vi "analyze graph array.vi"(7 "appended graphs":bool=TRUE, 9 "plot# per file":u16[](array[numeric])=[3, 1], 10 "column extension":string[](array[string])=["046", "044", "042"], 11 "graph file":cluster{"all rows":dbl[], "all rows":dbl[]}[](array[cluster])) -> (0 "total plot# per file":u16, 2 "reshuffled graph file":cluster{"all rows":dbl[], "all rows":dbl[]}[](array[cluster]), 3 "graph array summary":cluster{"index":u16, "length":u16}[](array[cluster]))   [LabVIEW 2025]
panel:
  out "valid":bool
  # "Find patterns of XY graphs\nInput: XY graphs from multiple data files. Each data file may have multiple plots. \nThe plots consists of singleX-multipleY and singleX-single Y and so forth.\n\n(1) Count number of the datafiles (same with the number of column extension)\n(2) Extract XY graphs of a single datafile, whose patterns are repeated for entire data files.\n(3) From the extracted XY graphs,  count number of rows of each xy-graph and find patterns\nin terms of the same number of rows (possibly due to graphs of same x-axis)."
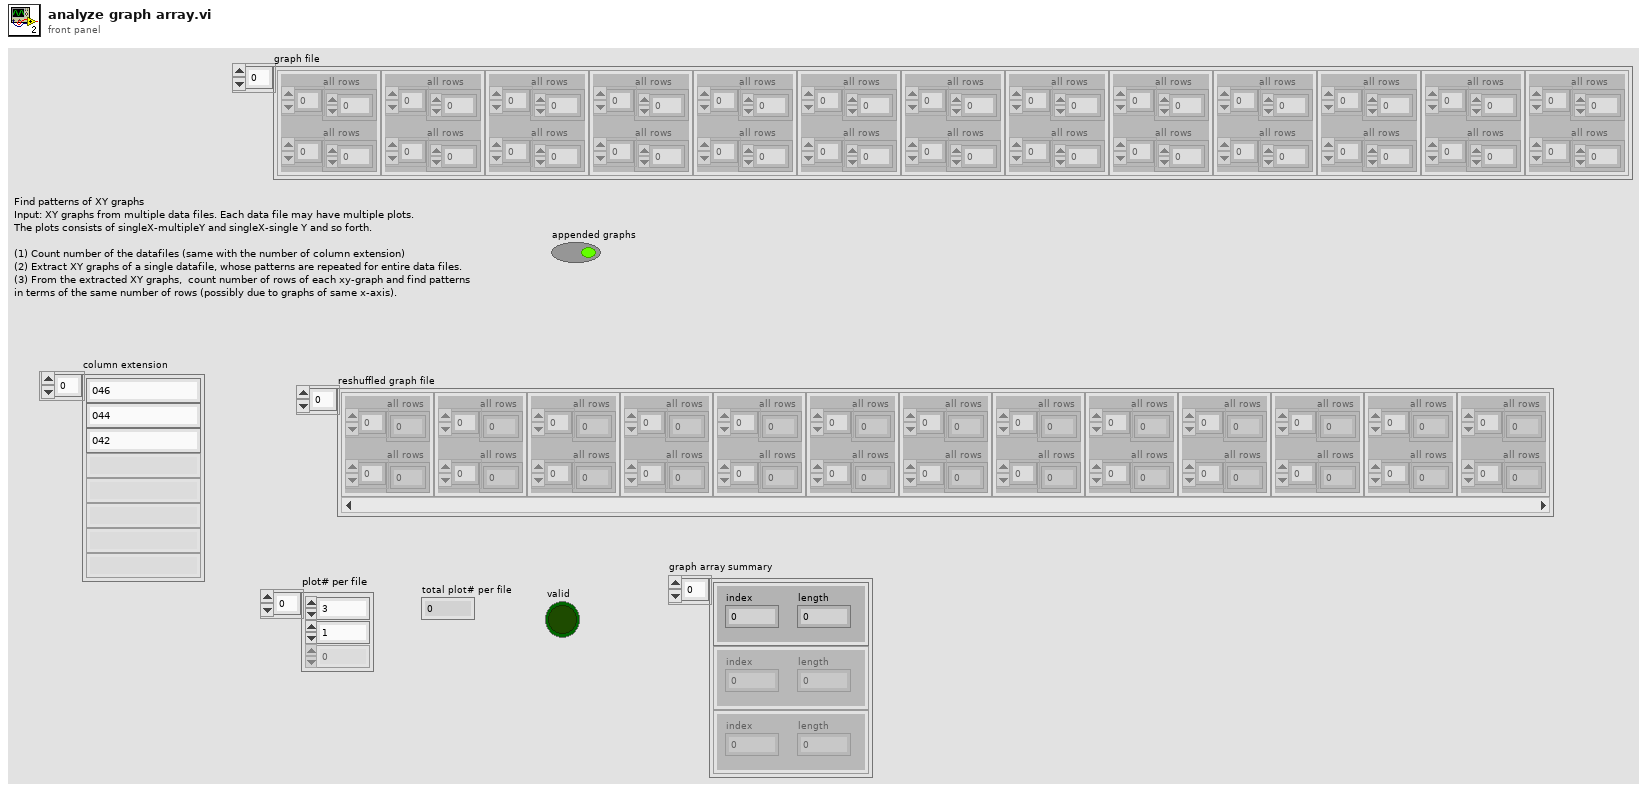
[diagram p1: front panel]
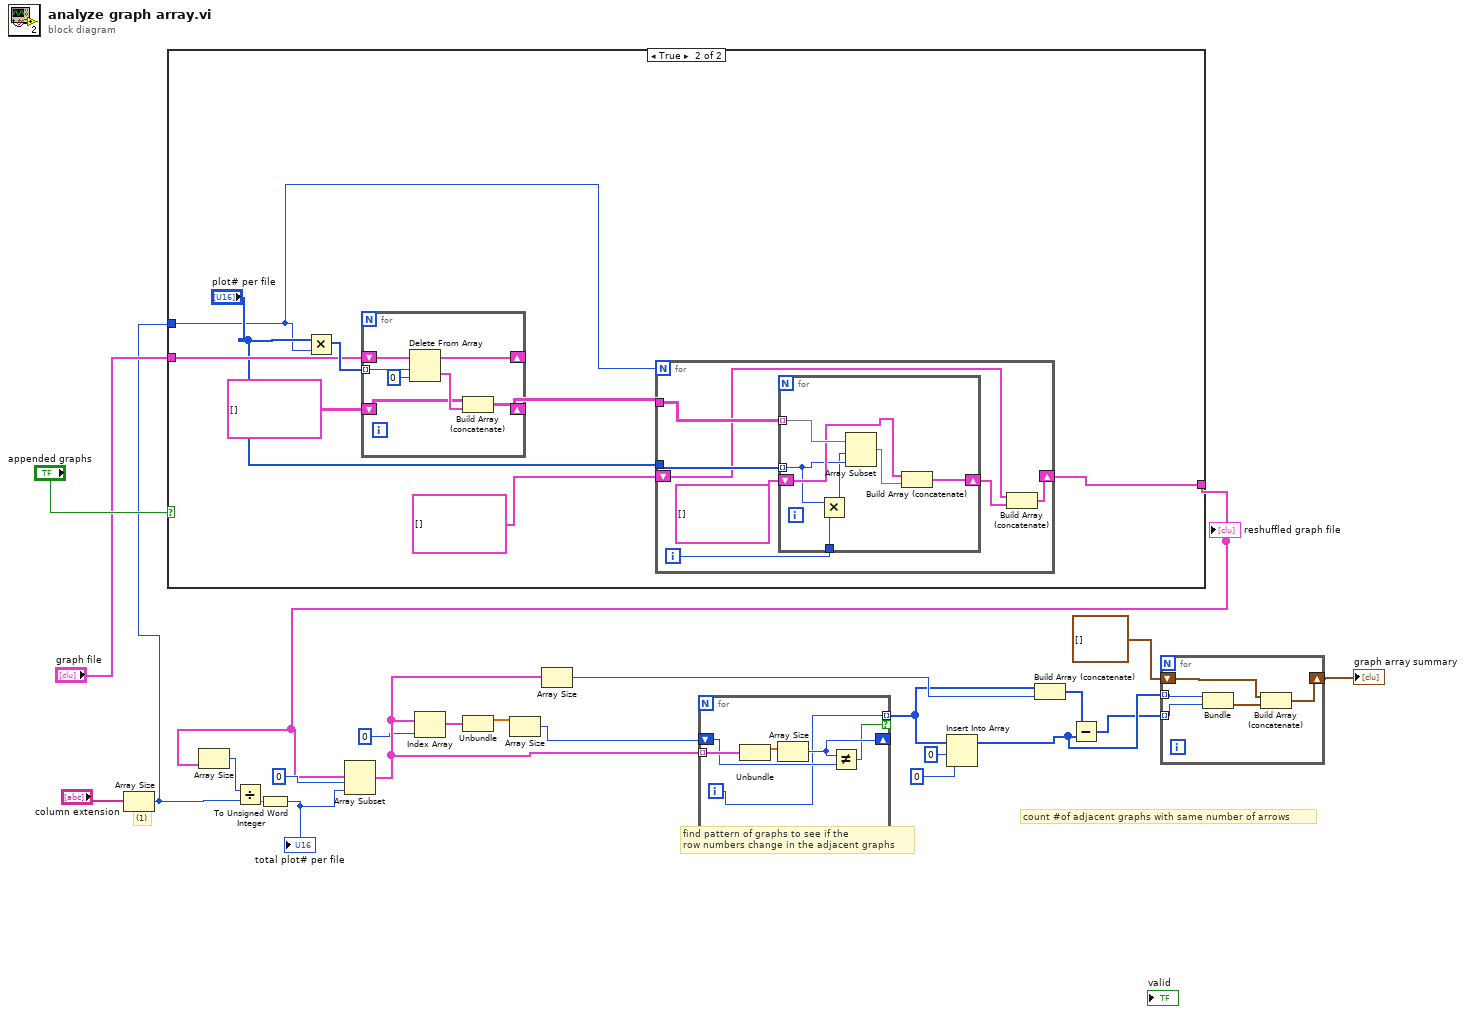
[diagram p0: block diagram]
diagram:
  # "(1)"
  # "count #of adjacent graphs with same number of arrows"
  # "find pattern of graphs to see if the\nrow numbers change in the adjacent graphs"
  n1 = Array Size(array="column extension") -> (size(s)=w2:i32)
  n2 = case shown="True" "appended graphs" {
    tunnel: "graph file" -> [w24 w29]
    tunnel: w2 -> [_ w25]
    tunnel: [w24 w28] -> w1
    frame False {
    }
    frame True {
      n3 = Multiply(x="plot# per file", y=w25) -> (x*y=w32:i32[])
      n4 = for {
        tunnel: w32 -> [w51] mode=indexing
        shift-right: [w52] -> _
        shift-left: w29 -> [w53]
        shift-right: [w49] -> w27
        shift-left: cluster{"all rows":dbl[], "all rows":dbl[]}[][] [] -> [w48]
        n5 = Delete From Array(array=w53, length=w51, index=0) -> (deleted portion=w50:cluster{"all rows":dbl[], "all rows":dbl[]}[], array with subset deleted=w52:cluster{"all rows":dbl[], "all rows":dbl[]}[])
        n6 = Build Array (concatenate)(w48, w50) -> (w49:cluster{"all rows":dbl[], "all rows":dbl[]}[][])
      }
      n7 = for {
        N: w25 -> [_]
        tunnel: "plot# per file" -> [w38]
        tunnel: w27 -> [w39]
        shift-right: [w34] -> w28
        shift-left: cluster{"all rows":dbl[], "all rows":dbl[]}[] [] -> [w35]
        i -> [w33]
        n8 = for {
          tunnel: w39 -> [w46] mode=indexing
          tunnel: w38 -> [w44] mode=indexing
          shift-right: [w40] -> w37
          shift-left: cluster{"all rows":dbl[], "all rows":dbl[]}[] [] -> [w45]
          tunnel: w33 -> [w43]
          n9 = Multiply(x=w44, y=w43) -> (x*y=w42:i32)
          n10 = Array Subset(array=w46, index=w42, length=w44) -> (w41:cluster{"all rows":dbl[], "all rows":dbl[]}[])
          n11 = Build Array (concatenate)(w45, w41) -> (w40:cluster{"all rows":dbl[], "all rows":dbl[]}[])
        }
        n12 = Build Array (concatenate)(w35, w37) -> (w34:cluster{"all rows":dbl[], "all rows":dbl[]}[])
      }
    }
  }
  "reshuffled graph file" <- w1
  n13 = Array Size(array=w1) -> (size(s)=w10:i32)
  n14 = Divide(x=w10, y=w2) -> (x/y=w7:dbl)
  n15 = To Unsigned Word Integer(number=w7) -> (unsigned 16bit integer=w4:u16)
  "total plot# per file" <- w4
  n16 = Array Subset(array=w1, index=0, length=w4) -> (w8:cluster{"all rows":dbl[], "all rows":dbl[]}[])
  n17 = Index Array(array=w8, index=0) -> (element=w13:cluster{"all rows":dbl[], "all rows":dbl[]})
  n18 = Unbundle(w13) -> ("all rows"=w12:dbl[])  [unwired: 1 out]
  n19 = Array Size(array=w12) -> (size(s)=w14:i32)
  n20 = Array Size(array=w8) -> (size(s)=w19:i32)
  n21 = for {
    tunnel: w8 -> [w59] mode=indexing
    shift-right: [w56] -> _
    shift-left: w14 -> [w57]
    tunnel: [w54] -> w17 mode=indexing if=w55
    i -> [w54]
    n22 = Unbundle(w59) -> ("all rows"=w58:dbl[])  [unwired: 1 out]
    n23 = Array Size(array=w58) -> (size(s)=w56:i32)
    n24 = Not Equal?(x=w56, y=w57) -> (x != y?=w55:bool)
  }
  n25 = Insert Into Array(array=w17, index=0, new element=0 ("new element/subarray")) -> (w21:i32[])
  n26 = Build Array (concatenate)(w17, w19) -> (w18:i32[])
  n27 = Subtract(x=w18, y=w21) -> (x-y=w20:i32[])
  n28 = for {
    tunnel: w20 -> [w63] mode=indexing
    tunnel: w21 -> [w64] mode=indexing
    shift-right: [w61] -> w23
    shift-left: cluster{i32, i32}[] [] -> [w60]
    n29 = Bundle(w64, w63) -> (w62:cluster{i32, i32})  [unwired: 1 in]
    n30 = Build Array (concatenate)(w60, w62) -> (w61:cluster{i32, i32}[])
  }
  "graph array summary" <- w23
